vi "ConvertAmplitude.vi"(10 "bits":i32, 11 "amplitude [0, 1]":dbl) -> (3 "generated amplitude [0, 2^(bits - 1) - 1]":dbl)   [LabVIEW 2016]
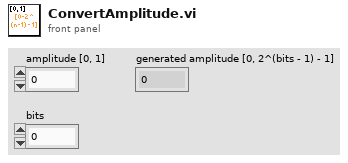
[diagram p1: front panel]
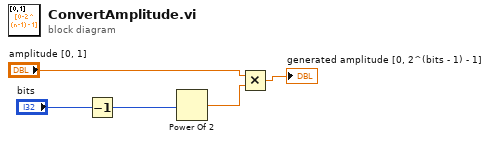
[diagram p0: block diagram]
diagram:
  n1 = Decrement(x="bits") -> (x-1=w5:i32)
  n2 = Power Of 2(x=w5) -> (2^x=w1:dbl)
  n3 = Multiply(x="amplitude [0, 1]", y=w1) -> (x*y=→"generated amplitude [0, 2^(bits - 1) - 1]":dbl)
